vi "Main UI.vi"(8 "error in (no error)":errorcluster, 10 "Initial Mouse (Demo)":refnum<class "Mouse.lvclass">) -> (0 "error out":errorcluster)   [LabVIEW 2020, in "App.lvlib" / "MazeUI.lvclass"]
uses:
  MazeUI.lvclass
  Maze/Maze/Maze.lvclass
  Maze/Mouse/Mouse.lvclass
  Mouse Type.ctl
  Demo/Demo Mouse/Demo Mouse.lvclass
  C:/dev/IlluminatedG/cc-maze/Maze/Mouse/Mouse.lvclass
  Maze/Direction.ctl
  <vilib>/Platform/browser.llb/Open URL in Default Browser (string).vi
  <vilib>/Utility/cursorutil.llb/Set Cursor (Icon Pict).vi
  Help UI.vi
  <vilib>/regexp/Match Regular Expression.xnode
  MazeFileIO/MazeFileIO.lvclass
  Maze/Maze.lvlib
  Maze/MazeGen/MazeGen.lvclass
panel:
  in  "Help Button":bool
  in  "Forums":bool
  in  "Configure Mouse":bool
  out "Mouse Name":string="Demo Mouse"
  in  "Run Speed":i32(slide)=100 scale=500.0..0.5
  out "Stepping":bool
  in  "Reset":bool
  in  "Step":bool
  out "Path":picture
  out "Walls":picture
  out "Actions":i32
  out "Mouse":refnum<class "Mouse.lvclass">
  in  "Stop":bool
  out "Running":bool
  out "Maze":refnum<class "Maze.lvclass">
  in  "Save":bool
  in  "Random":bool
  out "Maze":string
  in  "Load Maze":bool
  out "Status":string
  out "Mouse Author":string="Demo Mouse"
  in  "Load Mouse":bool
  in  "Start":bool
  out "Display":picture
  # "Summer of LabVIEW Maze Challenge"
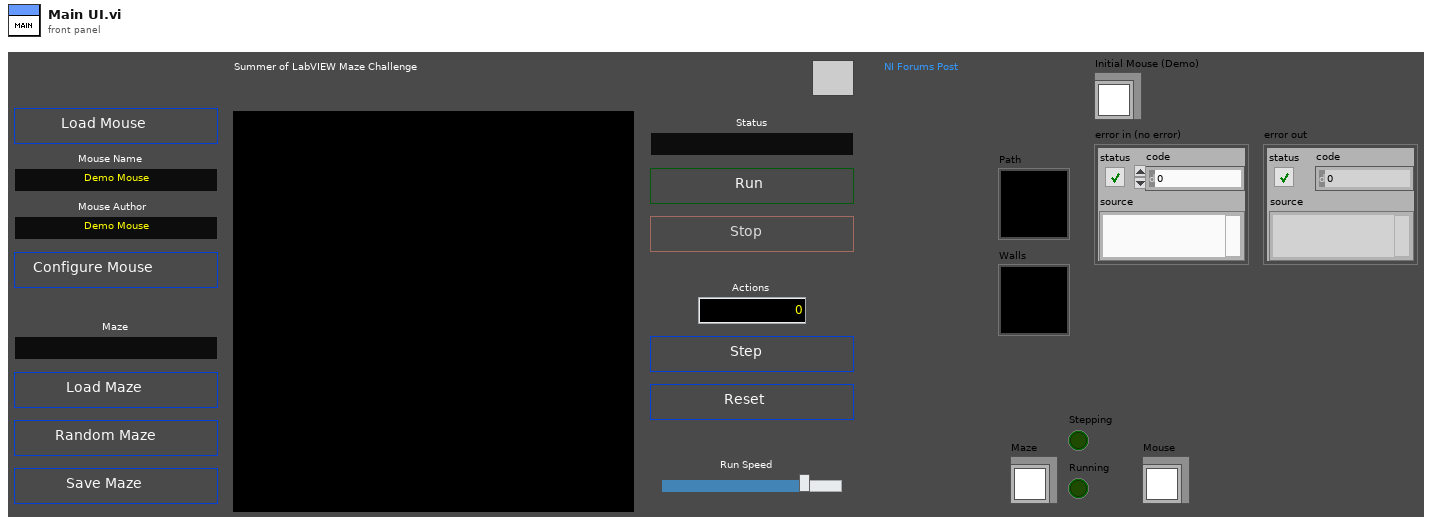
[diagram p1: front panel]
types:
  T1 = enum32{"Invalid", "Standard", "Closed", "Hidden", "Minimized", "Maximized"}
  T2 = enum8{"Enabled", "Disabled", "Disabled and Grayed Out"}
  T3 = typedef "App.lvlib/MazeUI.lvclass/Mouse Type.ctl" = enum16{"Instance", "Class Path", "LLB Path"}
  T4 = typedef "Maze.lvlib/Direction.ctl" = enum8{"East", "North", "West", "South"}
  T5 = typedef "Maze.lvlib/Position.ctl" = cluster{"S":i32, "E":i32}
  T6 = enum32{"Bad", "Idle", "Run top level", "Running"}
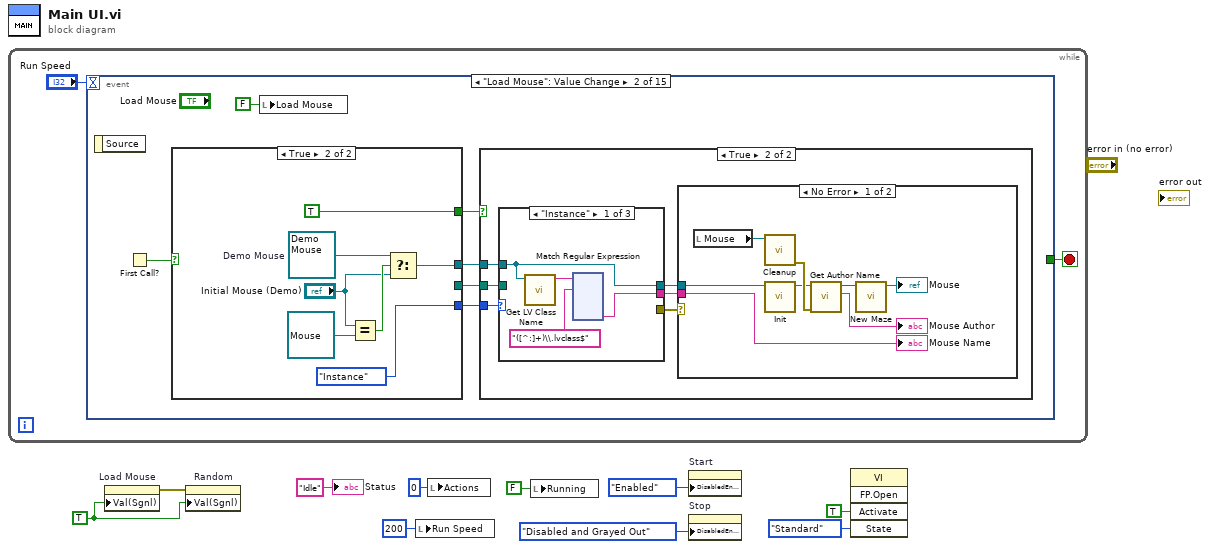
[diagram p0: block diagram]
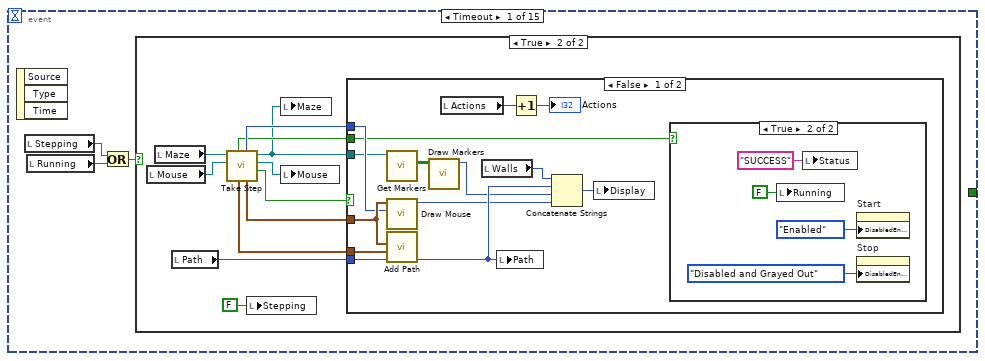
[diagram p2: hidden frame]
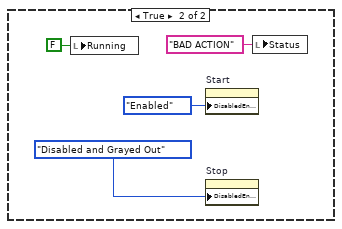
[diagram p5: hidden frame]
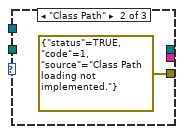
[diagram p7: hidden frame]
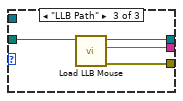
[diagram p8: hidden frame]
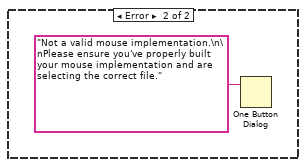
[diagram p9: hidden frame]
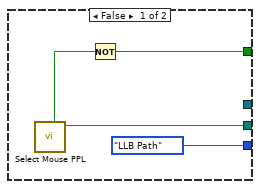
[diagram p10: hidden frame]
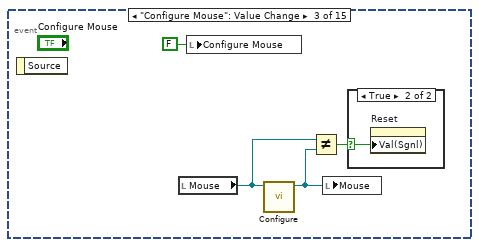
[diagram p11: hidden frame]
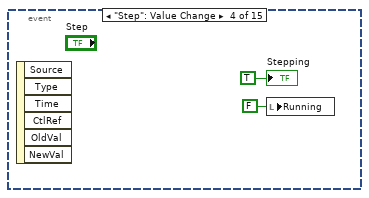
[diagram p13: hidden frame]
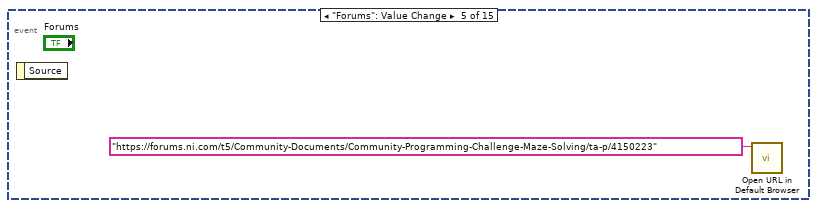
[diagram p14: hidden frame]
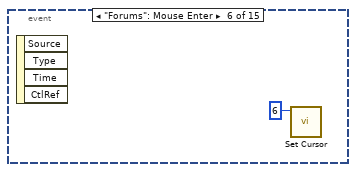
[diagram p15: hidden frame]
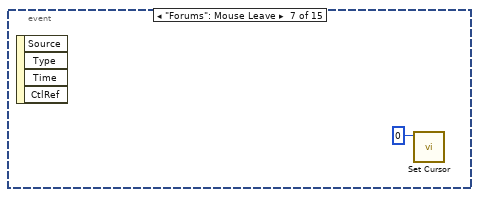
[diagram p16: hidden frame]
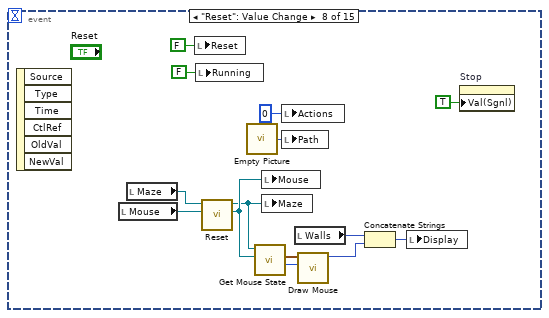
[diagram p17: hidden frame]
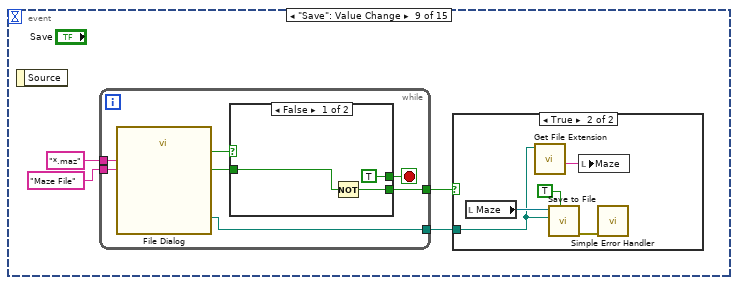
[diagram p18: hidden frame]
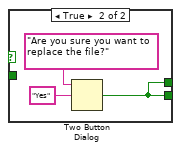
[diagram p20: hidden frame]
diagram:
  w4 = TRUE ("Value (Signaling)")
  n1 = while {
    stop <- w12 stop-if-true
    n2 = event shown="[1] \"Load Mouse\": Value Change" {
      selector: _ -> [_ _ _ _ _ _ _ _ _ _ _ _ _ _ _]
      dyn-events: _ -> [_ _ _ _ _ _ _ _ _ _ _ _ _ _ _]
      timeout: "Run Speed" -> [_ _ _ _ _ _ _ _ _ _ _ _ _ _ _]
      tunnel: [_ _ _ _ _ _ _ _ _ TRUE ("Discard?") _ _ _ _ _] -> w12
      event Timeout {
        n3 = event-data() -> ()  [unwired: 1 in, 3 out]
        n4 = local read "Stepping"() -> (w13:bool)
        n5 = local read "Running"() -> (w15:bool)
        n6 = Or(x=w13, y=w15) -> (x .or. y?=w14:bool)
        n7 = case shown="True" w14 {
          frame False {
          }
          frame True {
            n8 = local read "Mouse"() -> (w18:refnum<class "Mouse.lvclass">)
            n9 = local read "Maze"() -> (w26:refnum<class "Maze.lvclass">)
            n10 = local read "Path"() -> (w21:picture)
            n11 = call "Take Step.vi"("Mouse In"=w18, "Maze in"=w26) -> ("Bad Action?"=w25:bool, "Mouse"=w19:refnum<class "Mouse.lvclass">, "Maze"=w16:refnum<class "Maze.lvclass">, "New Position"=w23:T5, "Direction"=w24:T4, "Old Position"=w22:T5, "Goal?"=w17:bool)  [unwired: 2 in, 1 out]
            n12 = local write "Stepping"(FALSE ("Stepping")) -> ()
            n13 = local write "Maze"(w16) -> ()
            n14 = local write "Mouse"(w19) -> ()
            n15 = case shown="False" w25 {
              tunnel: w24 -> [w32 _]
              tunnel: w23 -> [w33 _]
              tunnel: w22 -> [w39 _]
              tunnel: w21 -> [w40 _]
              tunnel: w17 -> [w31 _]
              tunnel: w16 -> [w29 _]
              frame False {
                n16 = call "Get Markers.vi"("Maze in"=w29) -> ("Markers"=w28:bool[][])  [unwired: 8 in, 2 out]
                n17 = call "Draw Mouse.vi"("Direction"=w32, "Position"=w33) -> ("Picture"=w30:picture)  [unwired: 9 in]
                n18 = call "Add Path.vi"("Path In"=w40, "Old Position"=w39, "New Position"=w33) -> ("Path"=w37:picture)  [unwired: 8 in]
                n19 = call "Draw Markers.vi"("Markers"=w28) -> ("Picture"=w27:picture)  [unwired: 10 in]
                n20 = local read "Actions"() -> (w35:i32)
                n21 = local read "Walls"() -> (w38:picture)
                n22 = local write "Path"(w37) -> ()
                n23 = Increment(x=w35) -> (x+1=→"Actions":i32)
                n24 = Concatenate Strings(w38, w37, w27, w30) -> (w36:picture)
                n25 = local write "Display"(w36) -> ()
                n26 = case shown="True" w31 {
                  frame False {
                  }
                  frame True {
                    n27 = local write "Running"(FALSE ("Running")) -> ()
                    n28 = local write "Status"("SUCCESS" ("Status")) -> ()
                    n29 = property on="Start" class="Bool"("DisabledEnum"=T2."Enabled" ("Disabled")) -> ()  [unwired: 2 in, 2 out]
                    n30 = property on="Stop" class="Bool (strict)"("DisabledEnum"=T2."Disabled and Grayed Out" ("Disabled")) -> ()  [unwired: 2 in, 2 out]
                  }
                }
              }
              frame True {
                n31 = local write "Running"(FALSE ("Running")) -> ()
                n32 = property on="Start" class="Bool"("DisabledEnum"=T2."Enabled" ("Disabled")) -> ()  [unwired: 2 in, 2 out]
                n33 = property on="Stop" class="Bool (strict)"("DisabledEnum"=T2."Disabled and Grayed Out" ("Disabled")) -> ()  [unwired: 2 in, 2 out]
                n34 = local write "Status"("BAD ACTION" ("Status")) -> ()
              }
            }
          }
        }
      }
      event "Load Mouse": Value Change {
        n35 = event-data() -> ()  [unwired: 1 in, 1 out]
        n36 = First Call?() -> (First Call?: T/F=w53:bool)
        n37 = case shown="True" w53 {
          tunnel: [w196 TRUE] -> w52
          tunnel: [w198 _] -> w51
          tunnel: [Mouse_Type."LLB Path" ("Mouse Type") Mouse_Type."Instance" ("Mouse Type")] -> w50
          tunnel: [_ w200] -> w49
          frame False {
            n38 = call "Select Mouse PPL.vi"() -> ("selected path"=w198:path, "cancelled"=w197:bool)  [unwired: 10 in]
            n39 = Not(x=w197) -> (.not. x?=w196:bool)
          }
          frame True {
            w202 = refnum<class "Demo Mouse.lvclass"> refnum  # Demo Mouse
            n40 = Equal?(x="Initial Mouse (Demo)", y=refnum<class "Mouse.lvclass"> refnum ("x")) -> (x = y?=w203:bool)
            n41 = Select(t=w202, s=w203, f="Initial Mouse (Demo)") -> (s? t:f=w200:refnum<class "Mouse.lvclass">)
          }
        }
        n42 = local write "Load Mouse"(FALSE ("Load Mouse")) -> ()
        n43 = case shown="True" w52 {
          tunnel: w51 -> [_ w60]
          tunnel: w50 -> [_ w56]
          tunnel: w49 -> [_ w55]
          frame False {
          }
          frame True {
            n44 = case shown="\"Instance\"" w56 {
              tunnel: w60 -> [_ _ w185]
              tunnel: [w63 _ w184] -> w59
              tunnel: [w64 _ w183] -> w58
              tunnel: [_ errorcluster {"status"=TRUE, "code"=1, "source"="Class Path loading not implemented."} ("error out") w182] -> w57
              tunnel: w55 -> [w64 _ _]
              frame "Instance" {
                n45 = call <vilib>:"Get LV Class Name.vi"("object"=w64) -> ("class name"=w62:string)  [unwired: 9 in, 1 out]
                n46 = xnode "Match Regular Expression"("input string"=w62, "regular expression"="([^:]+)\\.lvclass$") -> ("submatch 1"=w63:string)  [unwired: 4 in, 5 out]
              }
              frame "Class Path" {
              }
              frame "LLB Path" {
                n47 = call "Load LLB Mouse.vi"("Mouse LLB"=w185) -> ("error out"=w182:errorcluster, "Name"=w184:string, "Mouse"=w183:refnum<class "Mouse.lvclass">)  [unwired: 8 in]
              }
            }
            n48 = case shown="No Error" w57 {
              tunnel: w58 -> [w189 _]
              tunnel: w59 -> [w188 _]
              frame No Error {
                n49 = local read "Mouse"() -> (w190:refnum<class "Mouse.lvclass">)
                n50 = call-dynamic "Cleanup.vi"("Mouse in"=w190) -> ("error out"=w193:errorcluster)  [unwired: 10 in]
                n51 = call-dynamic "Init.vi"("Mouse in"=w189) -> ("Mouse out"=w191:refnum<class "Mouse.lvclass">)  [unwired: 9 in, 1 out]
                n52 = call-dynamic "Get Author Name.vi"("error in (no error)"=w193, "Mouse in"=w191) -> ("Author"=→"Mouse Author":string, "Mouse out"=w187:refnum<class "Mouse.lvclass">)  [unwired: 7 in, 1 out]
                n53 = call-dynamic "New Maze.vi"("Mouse in"=w187) -> ("Mouse out"=→"Mouse":refnum<class "Mouse.lvclass">)  [unwired: 9 in, 1 out]
                "Mouse Name" <- w188
              }
              frame Error {
                n54 = One Button Dialog(message="Not a valid mouse implementation.\n\nPlease ensure you've properly built your mouse implementation and are selecting the correct file.") -> ()  [unwired: 1 in, 1 out]
              }
            }
          }
        }
      }
      event "Configure Mouse": Value Change {
        n55 = event-data() -> ()  [unwired: 1 in, 1 out]
        n56 = local read "Mouse"() -> (w207:refnum<class "Mouse.lvclass">)
        n57 = local write "Configure Mouse"(FALSE ("Configure Mouse")) -> ()
        n58 = call-dynamic "Configure.vi"("Mouse in"=w207) -> ("Mouse out"=w208:refnum<class "Mouse.lvclass">)  [unwired: 9 in, 1 out]
        n59 = Not Equal?(x=w207, y=w208) -> (x != y?=w206:bool)
        n60 = local write "Mouse"(w208) -> ()
        n61 = case shown="True" w206 {
          selector: w206 -> [_ w210]
          frame False {
          }
          frame True {
            n62 = property on="Reset" class="Bool (strict)"("Val(Sgnl)"=w210) -> ()  [unwired: 2 in, 2 out]
          }
        }
      }
      event "Step": Value Change {
        n63 = event-data() -> ()  [unwired: 1 in, 6 out]
        n64 = local write "Running"(FALSE ("Running")) -> ()
        "Stepping" <- TRUE ("Step")
      }
      event "Forums": Value Change {
        n65 = event-data() -> ()  [unwired: 1 in, 1 out]
        n66 = call-poly <vilib>:"Open URL in Default Browser.vi"("URL"="https://forums.ni.com/t5/Community-Documents/Community-Programming-Challenge-Maze-Solving/ta-p/4150223") -> ()  [unwired: 5 in, 2 out]
      }
      event "Forums": Mouse Enter {
        n67 = event-data() -> ()  [unwired: 1 in, 4 out]
        n68 = call-poly <vilib>:"Set Cursor.vi"("icon"=u16 6) -> ()  [unwired: 9 in, 2 out]
      }
      event "Forums": Mouse Leave {
        n69 = event-data() -> ()  [unwired: 1 in, 4 out]
        n70 = call-poly <vilib>:"Set Cursor.vi"("icon"=u16 0) -> ()  [unwired: 9 in, 2 out]
      }
      event "Reset": Value Change {
        n71 = event-data() -> ()  [unwired: 1 in, 6 out]
        n72 = local read "Mouse"() -> (w218:refnum<class "Mouse.lvclass">)
        n73 = local read "Maze"() -> (w228:refnum<class "Maze.lvclass">)
        n74 = local write "Reset"(FALSE ("Reset")) -> ()
        n75 = local write "Running"(FALSE ("Running")) -> ()
        n76 = call "Reset.vi"("Mouse In"=w218, "Maze in"=w228) -> ("Mouse"=w219:refnum<class "Mouse.lvclass">, "Maze out"=w217:refnum<class "Maze.lvclass">)  [unwired: 7 in, 1 out]
        n77 = call "Empty Picture"() -> ("empty picture"=w229:picture)
        n78 = call "Get Mouse State.vi"("Mouse"=w219, "Maze in"=w217) -> ("Direction"=w221:T4, "Position"=w222:T5)  [unwired: 6 in, 2 out]
        n79 = local write "Mouse"(w219) -> ()
        n80 = local write "Maze"(w217) -> ()
        n81 = local write "Actions"(0 ("Actions")) -> ()
        n82 = local write "Path"(w229) -> ()
        n83 = local read "Walls"() -> (w225:picture)
        n84 = call "Draw Mouse.vi"("Direction"=w221, "Position"=w222) -> ("Picture"=w224:picture)  [unwired: 9 in]
        n85 = Concatenate Strings(w225, w224) -> (w223:picture)
        n86 = local write "Display"(w223) -> ()
        n87 = property on="Stop" class="Bool (strict)"("Val(Sgnl)"=TRUE ("Value (Signaling)")) -> ()  [unwired: 2 in, 2 out]
      }
      event "Save": Value Change {
        n88 = event-data() -> ()  [unwired: 1 in, 1 out]
        n89 = while {
          tunnel: "*.maz" ("pattern (all files)") -> [w245]
          tunnel: "Maze File" ("pattern label") -> [w244]
          tunnel: [w241] -> w230
          tunnel: [w239] -> w231
          stop <- w240 stop-if-true
          n90 = call "File Dialog"("pattern (all files)"=w245, "pattern label"=w244) -> ("selected path"=w239:path, "exists"=w243:bool, "cancelled"=w242:bool)  [unwired: 10 in, 1 out]
          n91 = case shown="False" w243 {
            tunnel: w242 -> [w247 _]
            tunnel: [w248 w249] -> w241
            tunnel: [TRUE ("T button?") w249] -> w240
            frame False {
              n92 = Not(x=w247) -> (.not. x?=w248:bool)
            }
            frame True {
              n93 = Two Button Dialog(message="Are you sure you want to replace the file?", 2:"Yes" ("T button name (\"OK\")")) -> (T button?=w249:bool)  [unwired: 1 in]
            }
          }
        }
        n94 = case shown="True" w230 {
          tunnel: w231 -> [_ w235]
          frame False {
          }
          frame True {
            n95 = local read "Maze"() -> (w238:refnum<class "Maze.lvclass">)
            n96 = call <vilib>:"Get File Extension.vi"("file"=w235) -> ("filename without extension"=w234:string)  [unwired: 6 in, 4 out]
            n97 = call "Save to File.vi"("Replace if Exists? (F)"=TRUE, "Maze File Path (*.maz)"=w235, "Maze In"=w238) -> ("error out"=w236:errorcluster)  [unwired: 7 in, 1 out]
            n98 = local write "Maze"(w234) -> ()
            n99 = call <vilib>:"Simple Error Handler.vi"("error in (no error)"=w236) -> ()  [unwired: 4 in, 5 out]
          }
        }
      }
      event Panel Close {
        n100 = event-data() -> ()  [unwired: 1 in, 4 out]
        n101 = local read "Mouse"() -> (w252:refnum<class "Mouse.lvclass">)
        n102 = call-dynamic "Cleanup.vi"("Mouse in"=w252) -> ()  [unwired: 10 in, 1 out]
      }
      event "Help Button": Value Change {
        n103 = event-data() -> ()  [unwired: 1 in, 1 out]
        n104 = vi-ref "App.lvlib:MazeUI.lvclass:Help UI.vi"() -> (w259:refnum<vi>)
        n105 = property class="VI"(reference=w259) -> (reference out=w255:refnum<vi>, "Exec.State"=w258:T6)  [unwired: 1 in, 1 out]
        n106 = case shown="Default" w258 {
          tunnel: w255 -> [w260 w264]
          tunnel: [w260 w261] -> w254
          frame "Run top level", "Running" {
          }
          frame Default {
            n107 = invoke class="VI" method="Run VI"(reference=w264, "Wait until done"=FALSE ("Wait Until Done"), "Auto Dispose Ref"=TRUE ("Auto Dispose Reference")) -> (reference out=w261:refnum<vi>)  [unwired: 2 in, 4 out]
          }
        }
        n108 = invoke class="VI" method="FP.Open"(reference=w254, "Activate"=TRUE ("Activate?"), "State"=T1."Standard") -> ()  [unwired: 2 in, 5 out]
      }
      event "Load Maze": Value Change {
        n109 = event-data() -> ()  [unwired: 1 in, 1 out]
        n110 = call "File Dialog2"("pattern (all files)"="*.maz", "pattern label"="Maze File") -> ("selected path"=w268:path, "cancelled"=w265:bool)  [unwired: 10 in, 2 out]
        n111 = case shown="False" w265 {
          tunnel: w268 -> [w269 _]
          frame False {
            n112 = call "Load From File.vi"("Maze File Path (*.maz)"=w269) -> ("error out"=w270:errorcluster, "Maze"=w272:refnum<class "Maze.lvclass">)  [unwired: 9 in]
            n113 = case shown="No Error" w270 {
              selector: w270 -> [_ w282]
              tunnel: w272 -> [w277 _]
              tunnel: w269 -> [w276 _]
              frame No Error {
                n114 = local write "Maze"(w277) -> ()
                n115 = call <vilib>:"Get File Extension.vi"("file"=w276) -> ("filename without extension"=w275:string)  [unwired: 6 in, 4 out]
                n116 = call "Make Grid Overlay.vi"("Maze"=w277) -> ("Picture"=w280:picture)  [unwired: 10 in]
                n117 = call "Get Goal.vi"("Maze in"=w277) -> ("Goal"=w279:T5)  [unwired: 8 in, 2 out]
                n118 = call "Draw Goal.vi"("Position"=w279) -> ("Picture"=w278:picture)  [unwired: 10 in]
                n119 = local write "Maze"(w275) -> ()
                n120 = Concatenate Strings(w280, w278) -> (w281:picture)
                n121 = local read "Mouse"() -> (w274:refnum<class "Mouse.lvclass">)
                n122 = local write "Walls"(w281) -> ()
                n123 = call-dynamic "New Maze.vi"("Mouse in"=w274) -> ("Mouse out"=w273:refnum<class "Mouse.lvclass">)  [unwired: 9 in, 1 out]
                n124 = local write "Mouse"(w273) -> ()
              }
              frame Error {
                n125 = call <vilib>:"Simple Error Handler.vi"("error in (no error)"=w282) -> ()  [unwired: 4 in, 5 out]
              }
            }
            n126 = property on="Reset" class="Bool (strict)"("Val(Sgnl)"=TRUE ("Value (Signaling)")) -> ()  [unwired: 2 in, 2 out]
          }
          frame True {
          }
        }
      }
      event "Random": Value Change {
        n127 = event-data() -> ()  [unwired: 1 in, 1 out]
        n128 = First Call?() -> (First Call?: T/F=w283:bool)
        n129 = local write "Random"(FALSE ("Random")) -> ()
        n130 = case shown="False" w283 {
          tunnel: [w288 "Basic" ("Selected Level")] -> w285
          tunnel: [w287 FALSE ("Cancelled?")] -> w284
          frame False {
            n131 = call "Select Level UI.vi"() -> ("Cancelled?"=w287:bool, "Selected Level"=w288:string)  [unwired: 10 in]
          }
          frame True {
          }
        }
        n132 = case shown="False" w284 {
          tunnel: w285 -> [w293 _]
          frame False {
            w294 = 40 ("Height")
            n133 = call "Create Random Maze.vi"("Height (40)"=w294, "Width (40)"=w294, "Maze Level"=w293) -> ("Maze"=w295:refnum<class "Maze.lvclass">)  [unwired: 7 in, 1 out]
            "Maze" <- w295
            n134 = call "Make Grid Overlay.vi"("Maze"=w295) -> ("Picture"=w309:picture)  [unwired: 10 in]
            n135 = call "Get Goal.vi"("Maze in"=w295) -> ("Goal"=w306:T5)  [unwired: 8 in, 2 out]
            n136 = call "Get Start.vi"("Maze in"=w295) -> ("Start"=w308:T5)  [unwired: 8 in, 2 out]
            n137 = call "Draw Goal.vi"("Position"=w306) -> ("Picture"=w305:picture)  [unwired: 10 in]
            n138 = call "Draw Mouse.vi"("Direction"=Direction."East", "Position"=w308) -> ("Picture"=w301:picture)  [unwired: 9 in]
            n139 = Concatenate Strings(w309, w305) -> (w303:picture)
            "Walls" <- w303
            n140 = local write "Running"(FALSE ("Running")) -> ()
            n141 = local write "Status"("Idle" ("Status")) -> ()
            n142 = Concatenate Strings(w303, w301) -> (→"Display":picture)
            n143 = local read "Mouse"() -> (w292:refnum<class "Mouse.lvclass">)
            n144 = property on="Reset" class="Bool (strict)"("Val(Sgnl)"=TRUE ("Value (Signaling)")) -> ()  [unwired: 2 in, 2 out]
            n145 = call-dynamic "New Maze.vi"("Mouse in"=w292) -> ("Mouse out"=w291:refnum<class "Mouse.lvclass">)  [unwired: 9 in, 1 out]
            n146 = property on="Start" class="Bool"("DisabledEnum"=T2."Enabled" ("Disabled")) -> ()  [unwired: 2 in, 2 out]
            n147 = property on="Stop" class="Bool (strict)"("DisabledEnum"=T2."Disabled and Grayed Out" ("Disabled")) -> ()  [unwired: 2 in, 2 out]
            n148 = local write "Mouse"(w291) -> ()
            "Maze" <- "RANDOM" ("Maze")
          }
          frame True {
          }
        }
      }
      event "Start": Value Change {
        n149 = event-data() -> ()  [unwired: 1 in, 1 out]
        n150 = local read "Mouse"() -> (w313:refnum<class "Mouse.lvclass">)
        n151 = local read "Maze"() -> (w314:refnum<class "Maze.lvclass">)
        n152 = call "Empty Picture"() -> ("empty picture"=→"Path":picture)
        n153 = call "Reset.vi"("Mouse In"=w313, "Maze in"=w314) -> ("Mouse"=w312:refnum<class "Mouse.lvclass">, "Maze out"=w310:refnum<class "Maze.lvclass">)  [unwired: 7 in, 1 out]
        n154 = local write "Status"("Running" ("Status")) -> ()
        n155 = call-dynamic "Start.vi"("Mouse in"=w312) -> ("Mouse out"=w311:refnum<class "Mouse.lvclass">)  [unwired: 9 in, 1 out]
        n156 = local write "Maze"(w310) -> ()
        n157 = local write "Actions"(0 ("Actions")) -> ()
        n158 = local write "Mouse"(w311) -> ()
        n159 = property on="Start" class="Bool"("DisabledEnum"=T2."Disabled and Grayed Out" ("Disabled")) -> ()  [unwired: 2 in, 2 out]
        n160 = property on="Stop" class="Bool (strict)"("DisabledEnum"=T2."Enabled" ("Disabled")) -> ()  [unwired: 2 in, 2 out]
        "Running" <- TRUE ("Running")
      }
      event "Stop": Value Change {
        n161 = event-data() -> ()  [unwired: 1 in, 6 out]
        n162 = local write "Stop"(FALSE ("Stop")) -> ()
        n163 = local write "Running"(FALSE ("Running")) -> ()
        n164 = local write "Status"("Idle" ("Status")) -> ()
        n165 = property on="Start" class="Bool"("DisabledEnum"=T2."Enabled" ("Disabled")) -> ()  [unwired: 2 in, 2 out]
        n166 = property on="Stop" class="Bool (strict)"("DisabledEnum"=T2."Disabled and Grayed Out" ("Disabled")) -> ()  [unwired: 2 in, 2 out]
      }
    }
  }
  n167 = property on="Load Mouse" class="Bool (strict)"("Val(Sgnl)"=w4) -> (error out=w3:errorcluster)  [unwired: 2 in, 1 out]
  n168 = property on="Random" class="Bool (strict)"(error in=w3, "Val(Sgnl)"=w4) -> ()  [unwired: 1 in, 2 out]
  n169 = local write "Run Speed"(200 ("Run Speed")) -> ()
  n170 = local write "Actions"(0 ("Actions")) -> ()
  n171 = local write "Running"(FALSE ("Running")) -> ()
  n172 = property on="Start" class="Bool"("DisabledEnum"=T2."Enabled" ("Disabled")) -> ()  [unwired: 2 in, 2 out]
  n173 = property on="Stop" class="Bool (strict)"("DisabledEnum"=T2."Disabled and Grayed Out" ("Disabled")) -> ()  [unwired: 2 in, 2 out]
  n174 = invoke class="VI" method="FP.Open"("Activate"=TRUE ("Activate?"), "State"=T1."Standard") -> ()  [unwired: 3 in, 5 out]
  "Status" <- "Idle" ("Status")
